vi "LVUSBRH2_VISA_CMD_getrh_Q.vi"(8 "error in (no error)":errorcluster caption="error in(no errro)", 11 "VISA rssc":refnum<visa-resource-name>) -> (0 "error out":errorcluster, 1 "data[]":dbl[](array[numeric]), 3 "VISA rssc out":refnum<visa-resource-name>)   [LabVIEW 2020]
panel:
  out "recv string":string
  out "cmd string":string
  # "[0]温度\n[1]湿度"
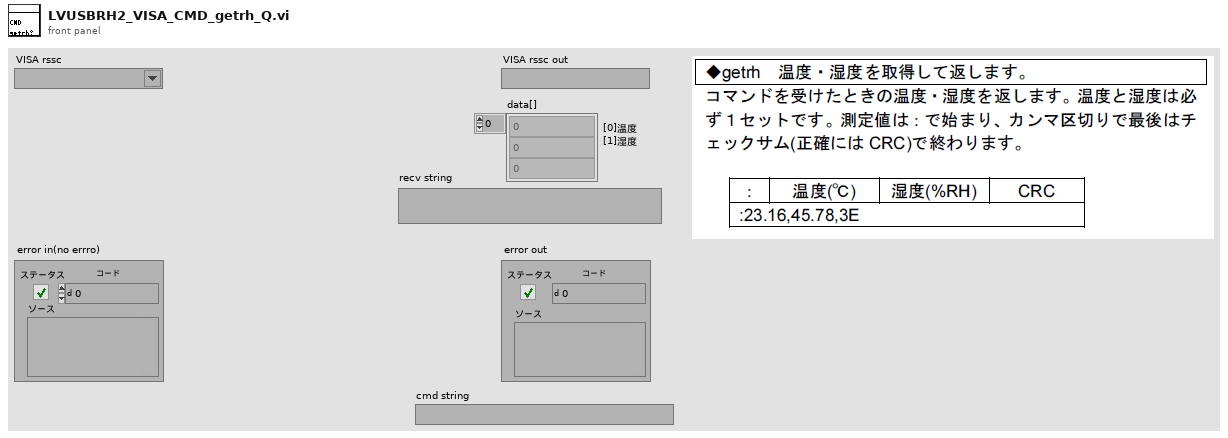
[diagram p1: front panel]
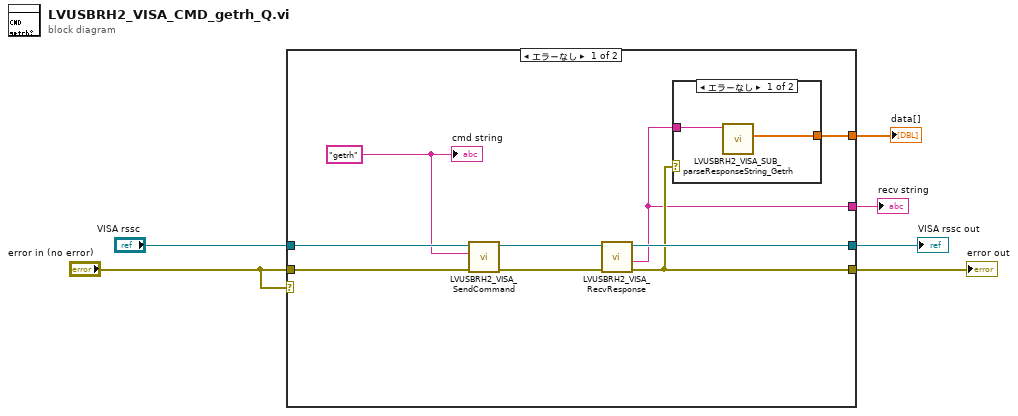
[diagram p0: block diagram]
diagram:
  n1 = case shown="エラーなし" "error in (no error)" {
    tunnel: "VISA rssc" -> [w15 w19]
    tunnel: [w12 w19] -> w5
    tunnel: "error in (no error)" -> [w14 w18]
    tunnel: [w9 w18] -> w4
    tunnel: [w8 _] -> w2
    tunnel: [w7 _] -> w1
    frame No Error {
      w11 = "getrh" ("形式文字列")
      n2 = call "LVUSBRH2_VISA_SendCommand.vi"("error in (no error)"=w14, "cmd string"=w11, "VISA rssc"=w15) -> ("error out"=w10:errorcluster, "VISA rssc out"=w13:refnum<visa-resource-name>)  [unwired: 7 in]
      n3 = call "LVUSBRH2_VISA_RecvResponse.vi"("error in (no error)"=w10, "VISA rssc"=w13) -> ("error out"=w9:errorcluster, "rcv string"=w8:string, "VISA rssc out"=w12:refnum<visa-resource-name>)  [unwired: 7 in]
      n4 = case shown="エラーなし" w9 {
        tunnel: w8 -> [w17 _]
        tunnel: [w16 _] -> w7
        frame No Error {
          n5 = call "LVUSBRH2_VISA_SUB_parseResponseString_Getrh.vi"("recv string"=w17) -> ("data[]"=w16:dbl[])  [unwired: 9 in, 1 out]
        }
        frame Error {
        }
      }
      "cmd string" <- w11
    }
    frame Error {
    }
  }
  "VISA rssc out" <- w5
  "error out" <- w4
  "recv string" <- w2
  "data[]" <- w1
